vi "wait_on_robots.vi"(8 "error in (no error)":errorcluster, 11 "Notifier in":refnum<notifier>) -> (0 "error out":errorcluster, 3 "Notifier out":refnum<notifier>)   [LabVIEW 2013]
uses:
  main_machine/type_defs/robotics_states.ctl
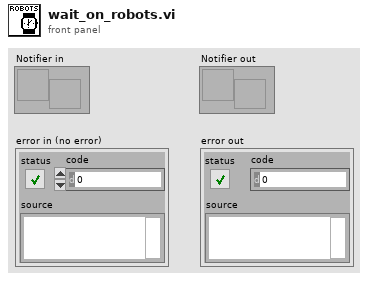
[diagram p1: front panel]
types:
  T1 = typedef "robotics_states.ctl" = enum16{"BUSY", "READY"}
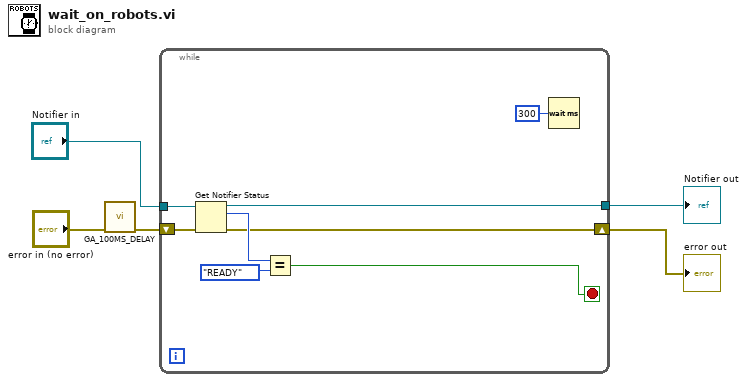
[diagram p0: block diagram]
diagram:
  n1 = call "GA_100MS_DELAY.vi"("Error IN"="error in (no error)") -> ("Error OUT"=w2:errorcluster)  [unwired: 10 in]
  n2 = while {
    tunnel: "Notifier in" -> [w13]
    shift-right: [w8] -> w1
    shift-left: w2 -> [w12]
    tunnel: [w7] -> w5
    stop <- w9 stop-if-true
    n3 = Get Notifier Status(notifier=w13, error in (no error)=w12) -> (notifier out=w7:refnum<notifier>, current notification=w11:T1, error out=w8:errorcluster)  [unwired: 2 out]
    n4 = Equal?(x=w11, y=robotics_states."READY" ("latest notification")) -> (x = y?=w9:bool)
    n5 = Wait (ms)(milliseconds to wait=u32 300) -> ()  [unwired: 1 out]
  }
  "error out" <- w1
  "Notifier out" <- w5
